vi "mupExpr Demo4.vi"() -> ()   [LabVIEW 2015]
uses:
  mupExpr/mupExpr.lvclass/mupExpr.ctl
  mupExpr/SetVarVal_Array.vi
  mupLib/mupEvalBulk.vi
  mupLib/mupSetVarValue_Array.vi
  mupLib/mupCheckError.vi
  mupLib/mupLibPath.vi
  <vilib>/Utility/error.llb/Error Cluster From Error Code.vi
  mupExpr/mupExpr.lvclass
panel:
  out "error out":errorcluster
  out "Results":dbl[](array[numeric]) format="%#_13g"
  out "Variable Names":string[](array[string])
  in  "Expression":string="a*x+b"
  in  "varValues":dbl[][](array[numeric])=[[1.0, 1.0, 1.0, 1.0], [1.0, 2.0, 3.0, 4.0], [5.0, 5.0, 5.0, 5.0]] format="%#_13g"
  # "Multiple variables, bulk mode"
  # "(one row per variable)"
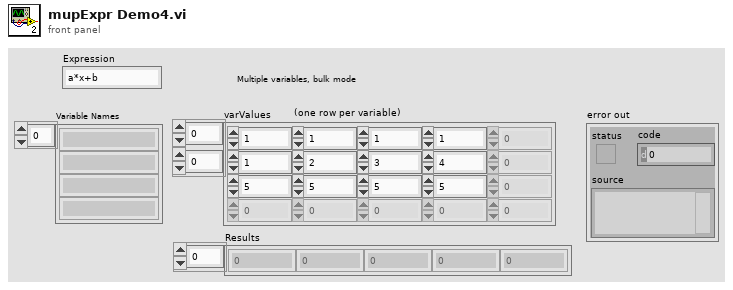
[diagram p1: front panel]
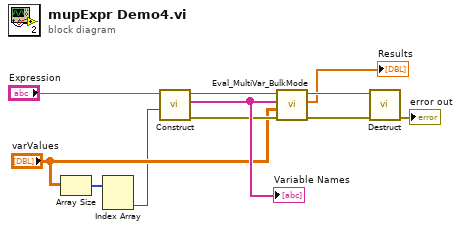
[diagram p0: block diagram]
diagram:
  n1 = Array Size(array="varValues") -> (size(s)=w2:i32[])
  n2 = Index Array(array=w2) -> (element #2=w1:i32)  [unwired: 2 in, 1 out]
  n3 = call "Construct.vi"("Bulk Size (1)"=w1, "Expression"="Expression") -> ("error out"=w7:errorcluster, "Variable Names"=w8:string[], "mupExpr out"=w6:refnum<data-value>)  [unwired: 7 in]
  "Variable Names" <- w8
  n4 = call "Eval_MultiVar_BulkMode.vi"("error in (no error)"=w7, "varValues"="varValues", "varNames"=w8, "mupExpr in"=w6) -> ("error out"=w9:errorcluster, "Result"=→"Results":dbl[], "mupExpr out"=w10:refnum<data-value>)  [unwired: 5 in]
  n5 = call "Destruct.vi"("error in (no error)"=w9, "mupExpr in"=w10) -> ("error out"=→"error out":errorcluster)  [unwired: 9 in]
